vi "niScope Sample Rate.vi"(0 "instrument handle":refnum<k15>, 11 "error in":errorcluster) -> (4 "instrument handle out":refnum<k15>, 8 "actual sample rate":dbl, 15 "error out":errorcluster)   [LabVIEW 2011]
doc: "Returns the effective sample rate, in samples per second, of the acquired waveform using the current configuration."
uses:
  niScope_32.dll
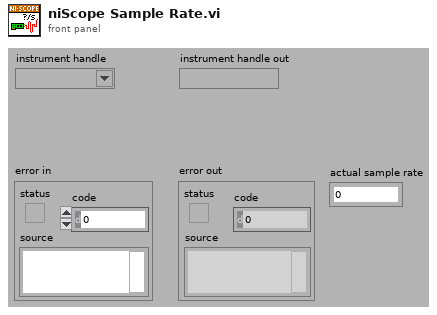
[diagram p1: front panel]
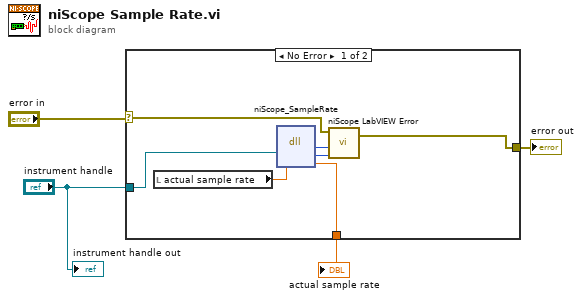
[diagram p0: block diagram]
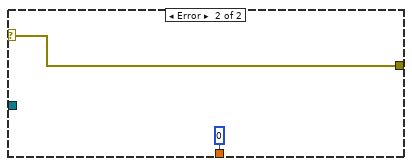
[diagram p2: hidden frame]
diagram:
  n1 = case shown="No Error" "error in" {
    selector: "error in" -> [w5 w12]
    tunnel: [w6 w12] -> w4
    tunnel: "instrument handle" -> [w11 _]
    tunnel: [w10 0 ("actual  record length")] -> w2
    frame No Error {
      n2 = local read "actual sample rate"() -> (w9:dbl)
      n3 = dll-call lib="niScope_*.*" fn="niScope_SampleRate"("instrument handle"=w11, "sampleRate"=w9) -> ("status"=w7:i32, "instrument handle"=w8:u32, "sampleRate"=w10:dbl)  [unwired: 3 in, 2 out]
      n4 = call <instrlib>:"niScope LabVIEW Error.vi"("instrument handle"=w8, "niScope error code (0)"=w7, "error in (no error)"=w5) -> ("error out"=w6:errorcluster)  [unwired: 2 in]
    }
    frame Error {
    }
  }
  "error out" <- w4
  "actual sample rate" <- w2
  "instrument handle out" <- "instrument handle"
